vi "COMSOL to Waveform Converter.vi"() -> ()   [LabVIEW 2013]
uses:
  <vilib>/Utility/file.llb/Read From Spreadsheet File (DBL).vi
  user.lib/Rearrange Array 1D Waveforms.vi
  <vilib>/Waveform/WDTFileIO.llb/ Write Waveforms to File (1D).vi
panel:
  in  "WFM":bool=TRUE
  out "all rows":dbl[][](array[numeric])
  out "COMSOL to Physical Index Map":u32[](array[numeric])
  in  "COMSOL to Physical Index Map File":path=path "C:/Users/plane/Dropbox/Research/MTA/DAQ VIs/Acoustic Data Toolbox/COMSOL to Waveform Converter/HPRF COMSOL to Physical Index Map.txt"
  out "Waveform Graph":waveform(dbl)[](graph)
  in  "Condition Signal":bool
  out "size(s)":i32
  in  "Right Padding Size":i32
  in  "Left Padding Size":i32
  out "Number of Channels":i32=6
  out "Samples per Channel":i32=100
  in  "1D Waveform Data File":path=path "C:/Users/plane/Desktop/COMSOL/Data/AllSignals_U_7_45_1e3.bin"
  in  "Process":bool
  in  "Load":bool
  in  "Save":bool
  in  "COMSOL CSV File":path=path "C:/Users/plane/Desktop/COMSOL/Data/AllSignals_U_7_45_1e3.csv"
  in  "Stop":bool
  # "1559"
  # "1559"
  # "Index = Sorted Index\nValue = Physical Index"
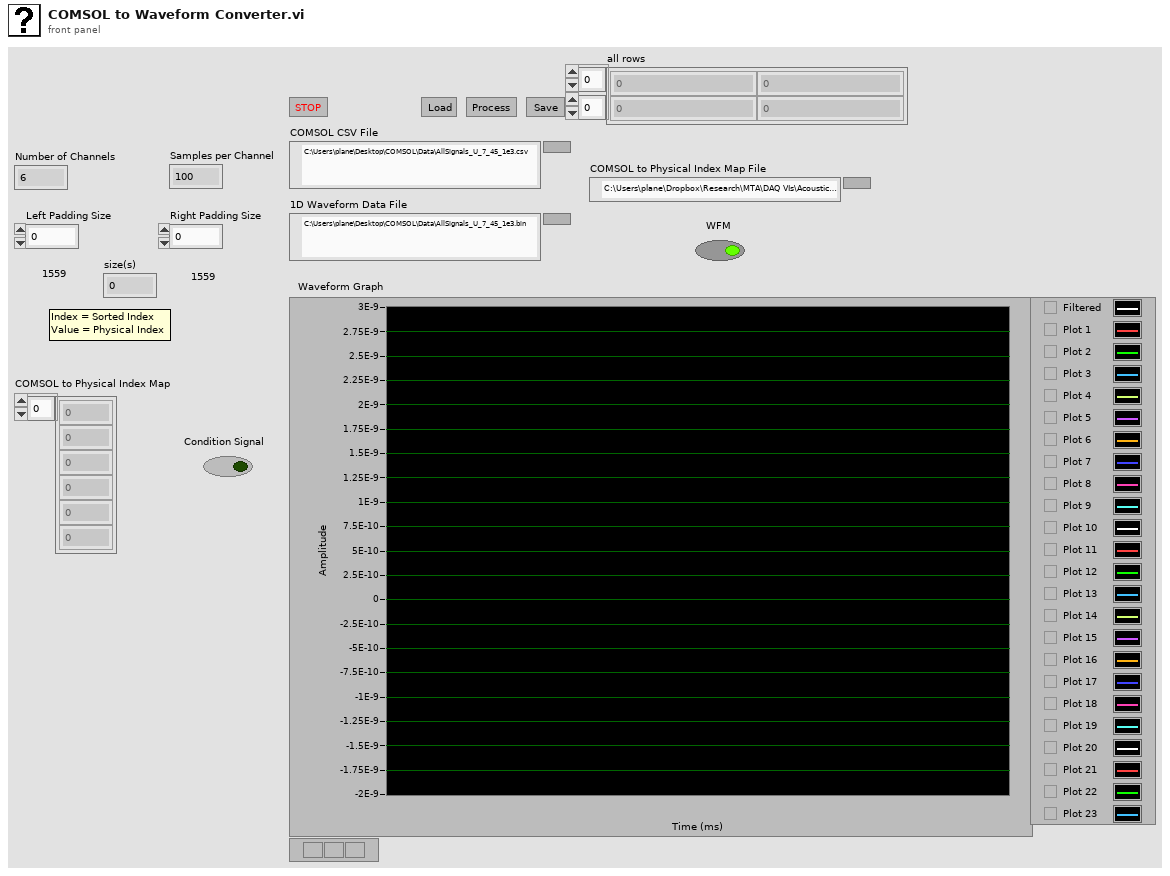
[diagram p1: front panel]
types:
  T1 = enum16{"big-endian, network order", "native, host order", "little-endian"}
  T2 = enum16{"open", "replace", "create", "open or create", "replace or create", "replace or create with confirmation"}
  T3 = enum32{"invalid app kind", "Development System", "Run Time System", "Student Edition", "Embedded LabVIEW", "Evaluation", "Custom"}
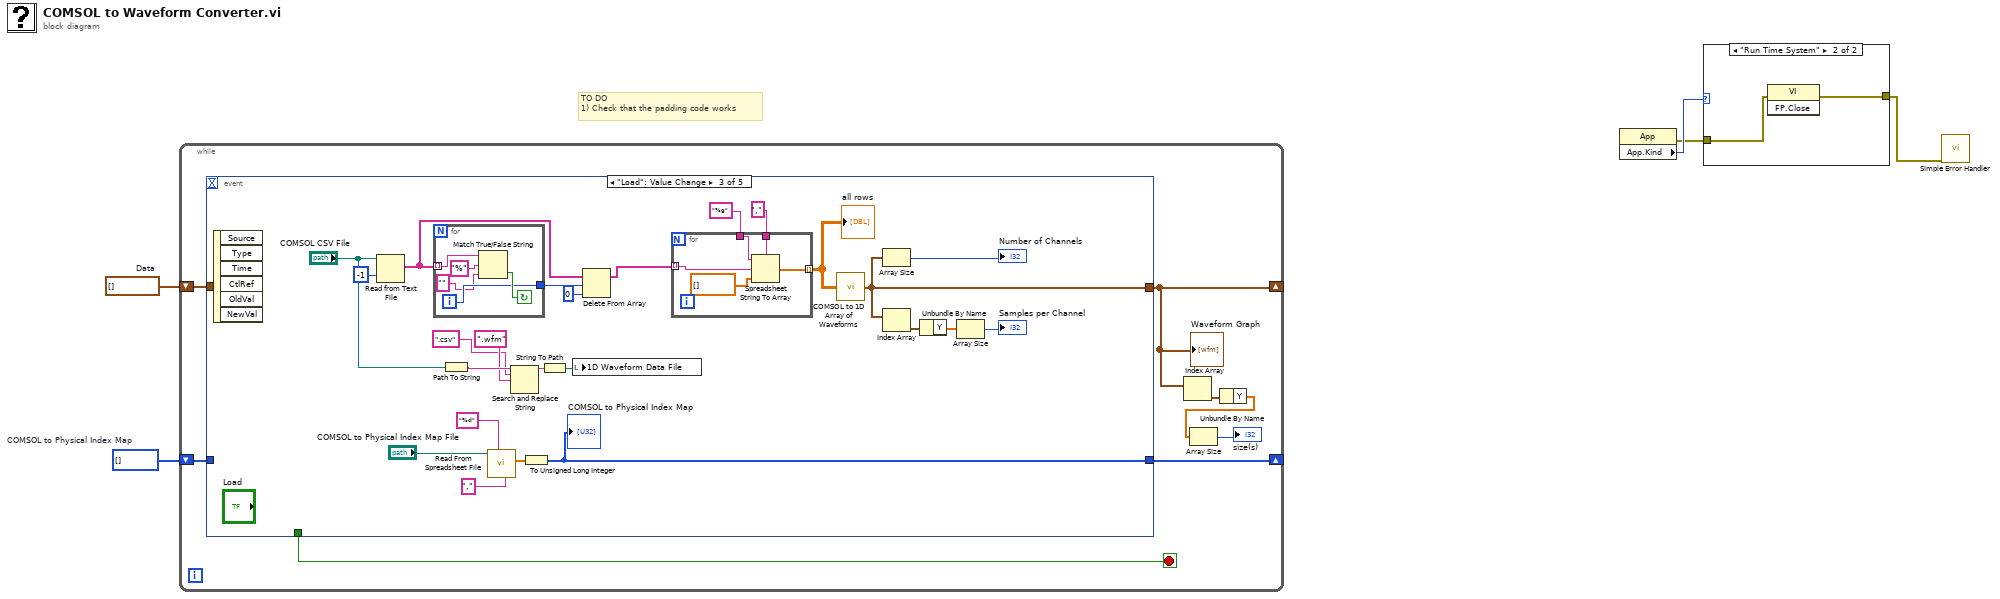
[diagram p0: block diagram]
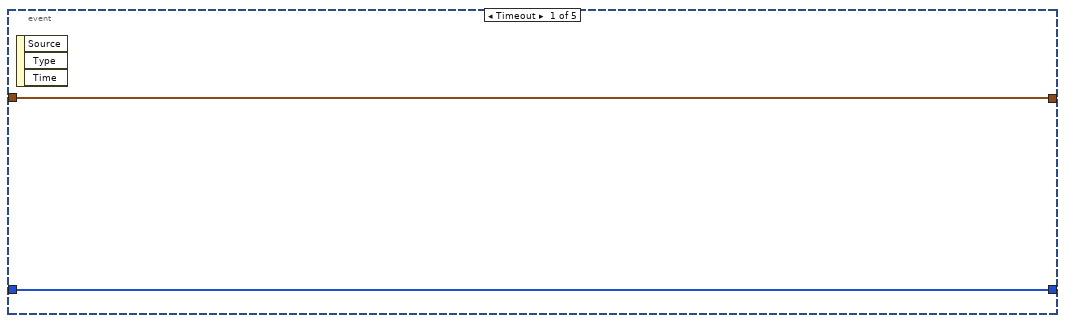
[diagram p2: hidden frame]
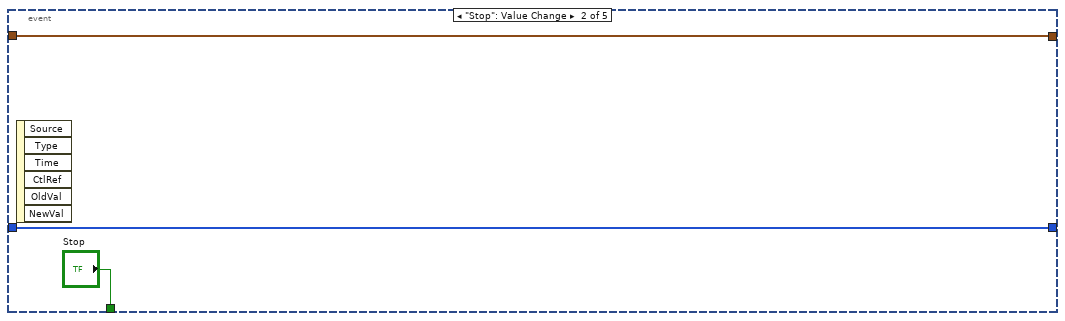
[diagram p3: hidden frame]
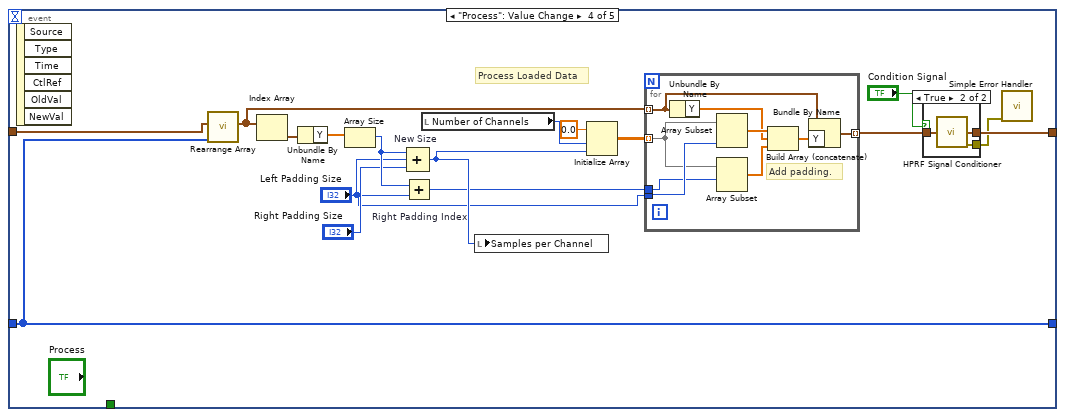
[diagram p4: hidden frame]
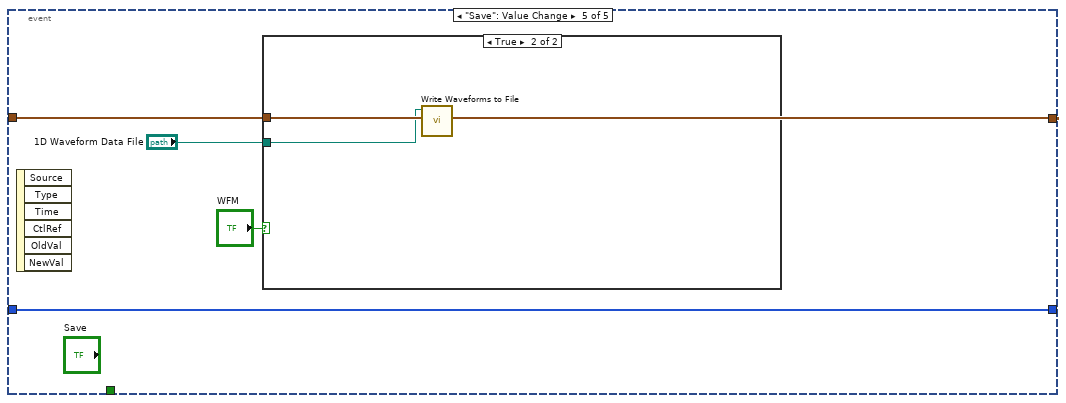
[diagram p6: hidden frame]
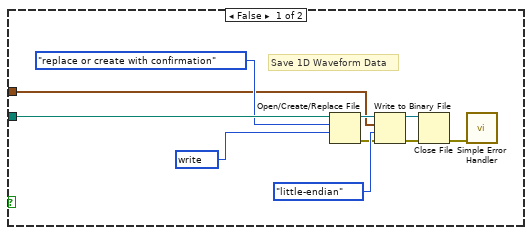
[diagram p7: hidden frame]
diagram:
  w1 = u32[] []  # COMSOL to Physical Index Map
  w2 = waveform(dbl)[] []  # Data
  # "TO DO\n1) Check that the padding code works"
  n1 = while {
    shift-right: [w8] -> _
    shift-left: w2 -> [w12]
    shift-right: [w7] -> _
    shift-left: w1 -> [w6]
    stop <- w13 stop-if-true
    n2 = event shown="[2] \"Load\": Value Change" {
      selector: _ -> [_ _ _ _ _]
      dyn-events: _ -> [_ _ _ _ _]
      timeout: _ -> [_ _ _ _ _]
      tunnel: [_ "Stop" _ _ _] -> w13
      tunnel: [w15 w17 w33 w56 w85] -> w8
      tunnel: w12 -> [w15 w17 _ w57 w85]
      tunnel: [w14 w16 w28 w53 w84] -> w7
      tunnel: w6 -> [w14 w16 _ w53 w84]
      event Timeout {
        n3 = event-data() -> ()  [unwired: 1 in, 3 out]
      }
      event "Stop": Value Change {
        n4 = event-data() -> ()  [unwired: 1 in, 6 out]
      }
      event "Load": Value Change {
        n5 = event-data() -> ()  [unwired: 1 in, 6 out]
        n6 = Read from Text File(file (use dialog)="COMSOL CSV File", count=-1) -> (text=w23:string[])  [unwired: 2 in, 3 out]
        n7 = for {
          tunnel: w23 -> [w46] mode=indexing
          tunnel: [w44] -> w20
          i -> [w44]
          stop <- w47 continue-if-true
          n8 = Match True/False String(2:"" ("false string"), 3:"%" ("true string"), 4:w46) -> (0:w47:bool)  [unwired: 1 out]
        }
        n9 = Path To String(path="COMSOL CSV File") -> (string=w41:string)
        n10 = call-poly <vilib>:"Read From Spreadsheet File.vi"("delimiter (\\t)"="," ("delimiter (\\t)"), "format (%.3f)"="%d", "file path (dialog if empty)"="COMSOL to Physical Index Map File") -> ("first row"=w29:dbl[])  [unwired: 4 in, 4 out]
        n11 = Search and Replace String(input string=w41, search string=".csv", replace string=".wfm" ("replace string (\"\")")) -> (result string=w40:string)  [unwired: 5 in, 3 out]
        n12 = To Unsigned Long Integer(number=w29) -> (unsigned 32bit integer=w28:u32[])
        "COMSOL to Physical Index Map" <- w28
        n13 = String To Path(string=w40) -> (path=w42:path)
        n14 = local write "1D Waveform Data File"(w42) -> ()
        n15 = Delete From Array(array=w23, length=w20, index=0) -> (array with subset deleted=w21:string[])  [unwired: 1 out]
        n16 = for {
          tunnel: "," ("delimiter (\\t)") -> [w52]
          tunnel: "%g" ("format (%.3f)") -> [w51]
          tunnel: w21 -> [w49] mode=indexing
          tunnel: [w48] -> w22 mode=indexing
          n17 = Spreadsheet String To Array(delimiter (Tab)=w52, format string=w51, spreadsheet string=w49, array type (2D Dbl)=dbl[] []) -> (array=w48:dbl[])
        }
        "all rows" <- w22
        n18 = call "COMSOL to 1D Array of Waveforms.vi"("COMSOL Data"=w22) -> ("1D Array of Waveforms"=w33:waveform(dbl)[])  [unwired: 14 in]
        n19 = Array Size(array=w33) -> (size(s)=→"Number of Channels":i32)
        n20 = Index Array(array=w33) -> (element=w37:waveform(dbl))  [unwired: 1 in]
        n21 = Unbundle By Name(w37) -> ("Y"=w36:dbl[])
        n22 = Array Size(array=w36) -> (size(s)=→"Samples per Channel":i32)
      }
      event "Process": Value Change {
        # "Process Loaded Data"
        n23 = event-data() -> ()  [unwired: 1 in, 6 out]
        n24 = call-poly "Rearrange Array.vi"("Index Map"=w53, "Array"=w57) -> ("Rearranged Array"=w66:waveform(dbl)[])  [unwired: 5 in]
        n25 = Index Array(array=w66) -> (element=w67:waveform(dbl))  [unwired: 1 in]
        n26 = Unbundle By Name(w67) -> ("Y"=w68:dbl[])
        n27 = Array Size(array=w68) -> (size(s)=w65:i32)
        n28 = Add "Right Padding Index"(x=w65, y="Left Padding Size") -> (x+y=w61:i32)
        n29 = Compound Arithmetic op=ADD "New Size"(w65, "Left Padding Size", "Right Padding Size") -> (w64:i32)
        n30 = local read "Number of Channels"() -> (w59:i32)
        n31 = local write "Samples per Channel"(w64) -> ()
        n32 = Initialize Array(0.0 ("element"), w59, w64) -> (w60:dbl[][])
        n33 = for {
          tunnel: w66 -> [w76] mode=indexing
          tunnel: "Left Padding Size" -> [w82]
          tunnel: w61 -> [w81]
          tunnel: w60 -> [w78] mode=indexing
          tunnel: [w75] -> w69 mode=indexing
          # "Add padding."
          n34 = Unbundle By Name(w76) -> ("Y"=w77:dbl[])
          n35 = Array Subset(array=w78, length=w82) -> (w80:dbl[])  [unwired: 1 in]
          n36 = Array Subset(array=w78, index=w81) -> (w79:dbl[])  [unwired: 1 in]
          n37 = Build Array (concatenate)(w80, w77, w79) -> (w74:dbl[])
          n38 = Bundle By Name(cluster=w76, "Y"=w74) -> (w75:waveform(dbl))
        }
        n39 = case shown="True" "Condition Signal" {
          tunnel: w69 -> [w70 w73]
          tunnel: [w70 w72] -> w56
          tunnel: [_ w71] -> w54
          frame False {
          }
          frame True {
            n40 = call "HPRF Signal Conditioner.vi"("Signals"=w73) -> ("Condintioned Signals"=w72:waveform(dbl)[], "error out"=w71:errorcluster)  [unwired: 13 in]
          }
        }
        n41 = call <vilib>:"Simple Error Handler.vi"("error in (no error)"=w54) -> ()  [unwired: 4 in, 5 out]
      }
      event "Save": Value Change {
        n42 = event-data() -> ()  [unwired: 1 in, 6 out]
        n43 = case shown="True" "WFM" {
          tunnel: "1D Waveform Data File" -> [w96 w97]
          tunnel: w85 -> [w87 w98]
          frame False {
            w92 = u32 1073741824 items=["read"=2147483648, "write"=1073741824, "read & write"=3221225472, "execute"=536870912, "all"=268435456] ("desired access (read & write)")
            # "Save 1D Waveform Data"
            n44 = Open/Create/Replace File(file path (use dialog)=w96, operation (0:open)=T2."replace or create with confirmation", access (0:read/write)=w92) -> (refnum out=w93:refnum<file>, error out=w94:errorcluster)  [unwired: 3 in, 1 out]
            n45 = Write to Binary File(file (use dialog)=w93, data=w87, error in=w94, 9:T1."little-endian" ("byte order (0:big-endian, network order)")) -> (refnum out=w89:refnum<file>, error out=w90:errorcluster)  [unwired: 2 in, 1 out]
            n46 = Close File(refnum=w89, error in=w90) -> (error out=w88:errorcluster)  [unwired: 1 out]
            n47 = call <vilib>:"Simple Error Handler.vi"("error in (no error)"=w88) -> ()  [unwired: 4 in, 5 out]
          }
          frame True {
            n48 = call-poly <vilib>:"Write Waveforms to File.vi"("waveform array"=w98, "file path (dialog if empty)"=w97) -> ()  [unwired: 8 in, 2 out]
          }
        }
      }
    }
    "Waveform Graph" <- w8
    n49 = Index Array(array=w8) -> (element=w11:waveform(dbl))  [unwired: 1 in]
    n50 = Unbundle By Name(w11) -> ("Y"=w9:dbl[])
    n51 = Array Size(array=w9) -> (size(s)=→"size(s)":i32)
  }
  n52 = property class="App"() -> (error out=w4:errorcluster, "App.Kind"=w5:T3)  [unwired: 2 in, 1 out]
  n53 = case shown="\"Run Time System\"" w5 {
    tunnel: w4 -> [w99 w101]
    tunnel: [w99 w100] -> w3
    frame Default {
    }
    frame "Run Time System" {
      n54 = invoke class="VI" method="FP.Close"(error in=w101) -> (error out=w100:errorcluster)  [unwired: 2 in, 2 out]
    }
  }
  n55 = call <vilib>:"Simple Error Handler.vi"("error in (no error)"=w3) -> ()  [unwired: 4 in, 5 out]
